vi "Get PMU Configuration2.vi"(8 "error in (no error)":errorcluster, 10 "PMU Index":i32, 11 "Pseudo PDC ID":i32) -> (0 "error out":errorcluster, 3 "PMU Configuration":T1)   [LabVIEW 2018, in "S3DK.lvlib" / "PMU Recorder Light.lvlib" / "Statnett C37.118 DLL.lvclass"]
uses:
  Statnett C37.118 DLL.lvclass
  c37118-dll/C37118-DLL.lvlib
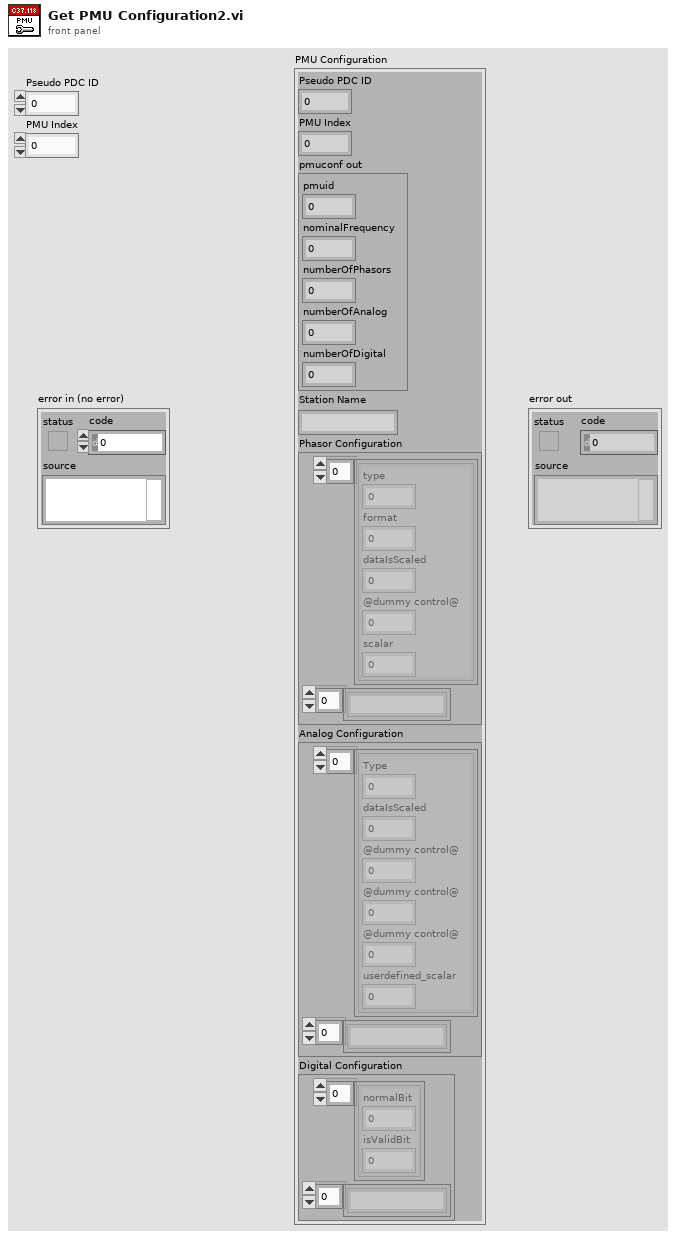
[diagram p1: front panel]
types:
  T1 = cluster{"Pseudo PDC ID":i32, "PMU Index":i32, "pmuconf out":cluster{"pmuid":i32, "nominalFrequency":sgl, "numberOfPhasors":i32, "numberOfAnalog":i32, "numberOfDigital":i32}, "Station Name":string, "Phasor Configuration":cluster{cluster{"type":u8, "format":u8, "dataIsScaled":u8, "@dummy control@":i8, "scalar":sgl}[], string[]}, "Analog Configuration":cluster{cluster{"Type":i32, "dataIsScaled":u8, "@dummy control@":i8, "@dummy control@":i8, "@dummy control@":i8, "userdefined_scalar":sgl}[], string[]}, "Digital Configuration":cluster{cluster{"normalBit":u8, "isValidBit":u8}[], string[]}}
  T2 = cluster{"pmuid":i32, "nominalFrequency":sgl, "numberOfPhasors":i32, "numberOfAnalog":i32, "numberOfDigital":i32}
  T3 = cluster{cluster{"normalBit":u8, "isValidBit":u8}[], string[]}
  T4 = cluster{cluster{"Type":i32, "dataIsScaled":u8, "@dummy control@":i8, "@dummy control@":i8, "@dummy control@":i8, "userdefined_scalar":sgl}[], string[]}
  T5 = cluster{cluster{"type":u8, "format":u8, "dataIsScaled":u8, "@dummy control@":i8, "scalar":sgl}[], string[]}
  T6 = cluster{"Pseudo PDC ID":i32, "PMU Index":i32, "PMU Configuration":cluster{"pmuid":i32, "nominalFrequency":sgl, "numberOfPhasors":i32, "numberOfAnalog":i32, "numberOfDigital":i32}, "Station Name":string, "Phasor Configuration":cluster{cluster{"type":u8, "format":u8, "dataIsScaled":u8, "@dummy control@":i8, "scalar":sgl}[], string[]}, "Analog Configuration":cluster{cluster{"Type":i32, "dataIsScaled":u8, "@dummy control@":i8, "@dummy control@":i8, "@dummy control@":i8, "userdefined_scalar":sgl}[], string[]}, "Digital Configuration":cluster{cluster{"normalBit":u8, "isValidBit":u8}[], string[]}}
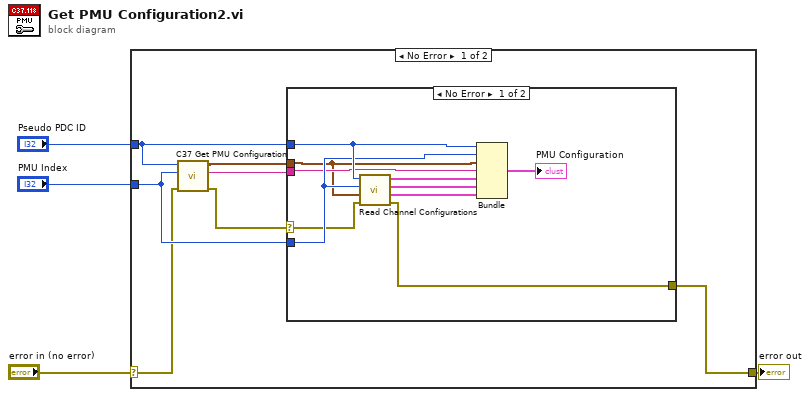
[diagram p0: block diagram]
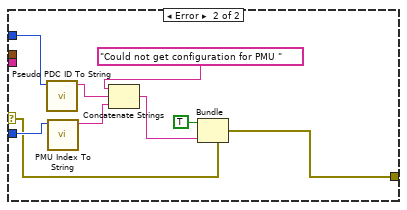
[diagram p2: hidden frame]
diagram:
  n1 = case shown="No Error" "error in (no error)" {
    selector: "error in (no error)" -> [w5 w31]
    tunnel: [w11 w31] -> w3
    tunnel: "Pseudo PDC ID" -> [w10 _]
    tunnel: "PMU Index" -> [w9 _]
    frame No Error {
      n2 = call "C37 Get PMU Configuration.vi"("error in (no error)"=w5, "PMU Index"=w9, "Pseudo PDC ID"=w10) -> ("error out"=w6:errorcluster, "Station Name"=w7:string, "PMU Configuration"=w8:T2)  [unwired: 6 in]
      n3 = case shown="No Error" w6 {
        selector: w6 -> [w14 w22]
        tunnel: w7 -> [w15 _]
        tunnel: w8 -> [w12 _]
        tunnel: w9 -> [w16 w26]
        tunnel: [w21 w27] -> w11
        tunnel: w10 -> [w17 w25]
        frame No Error {
          n4 = call "Read Channel Configurations.vi"("error in (no error)"=w14, "PMU Configuration"=w12, "PMU Index"=w16, "Pseudo PDC ID"=w17) -> ("error out"=w21:errorcluster, "Digital Configuration"=w18:T3, "Analog Configuration"=w19:T4, "Phasor Configuration"=w20:T5)  [unwired: 4 in]
          n5 = Bundle("Pseudo PDC ID"=w17, "PMU Index"=w16, "PMU Configuration"=w12, "Station Name"=w15, "Phasor Configuration"=w20, "Analog Configuration"=w19, "Digital Configuration"=w18) -> (→"PMU Configuration":T6)  [unwired: 1 in]
        }
        frame Error {
          n6 = call "Pseudo PDC ID To String.vi"("Pseudo PDC ID"=w25) -> ("String"=w24:string)  [unwired: 10 in]
          n7 = call "PMU Index To String.vi"("PMU Index"=w26) -> ("String"=w23:string)  [unwired: 10 in]
          n8 = Concatenate Strings("Could not get configuration for PMU " ("source"), w24, w23) -> (w28:string)
          n9 = Bundle(cluster=w22, "status"=TRUE, "source"=w28) -> (w27:errorcluster)  [unwired: 1 in]
        }
      }
    }
    frame Error {
    }
  }
  "error out" <- w3
